vi "AI Acquisition Setup.vi"(11 "Analog Input Data":T1) -> (0 "error out":errorcluster, 3 "Refnum out":refnum<k21>)   [LabVIEW 2021]
doc: "This VI receives the cluster data necessary to setup and start the DAQmx analog input data acquisition."
uses:
  <vilib>/DAQmx/create/channels.llb/DAQmx Create Channel (AI-Voltage-Basic).vi
  <vilib>/DAQmx/configure/timing.llb/DAQmx Timing (Sample Clock).vi
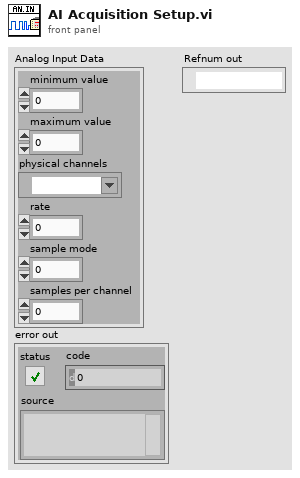
[diagram p1: front panel]
types:
  T1 = cluster{"minimum value":dbl, "maximum value":dbl, "physical channels":tag, "rate":dbl, "sample mode":i32, "samples per channel":i32}
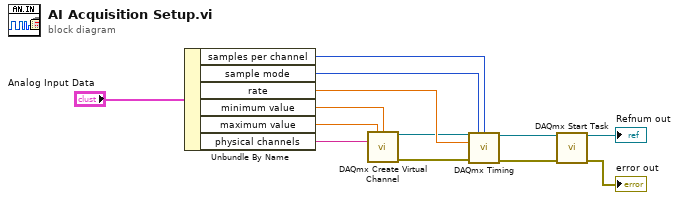
[diagram p0: block diagram]
diagram:
  n1 = Unbundle By Name("Analog Input Data") -> ("samples per channel"=w13:i32, "sample mode"=w12:i32, "rate"=w11:dbl, "minimum value"=w10:dbl, "maximum value"=w9:dbl, "physical channels"=w8:tag)
  n2 = call-poly <vilib>:"DAQmx Create Virtual Channel.vi"("maximum value"=w9, "minimum value"=w10, "physical channels"=w8) -> ("task out"=w1:refnum<k21>, "error out"=w4:errorcluster)  [unwired: 11 in]
  n3 = call-poly <vilib>:"DAQmx Timing.vi"("task/channels in"=w1, "sample mode"=w12, "samples per channel"=w13, "rate"=w11, "error in"=w4) -> ("task out"=w2:refnum<k21>, "error out"=w5:errorcluster)  [unwired: 9 in]
  n4 = call <vilib>:"DAQmx Start Task.vi"("task/channels in"=w2, "error in"=w5) -> ("task out"=→"Refnum out":refnum<k21>, "error out"=→"error out":errorcluster)  [unwired: 12 in]
